vi "Add PV (NT Enum (Index & Choices)).vi"(6 "initial timestamp":timestamp, 7 "PV name":string, 8 "error in (no error)":errorcluster, 9 "initial choices":string[](array[string]), 10 "initial index":u16(ring), 11 "Server in":refnum<class "Server.lvclass">) -> (0 "error out":errorcluster, 1 "choices out":string[](array[string]), 2 "value out":u16, 3 "Server out":refnum<class "Server.lvclass">, 4 "timestamp out":timestamp)   [LabVIEW 2020, in "PV Access.lvlib" / "PVA Server.lvlib" / "Server.lvclass"]
uses:
  Server.lvclass
  PV Data/NT Enum/NT Enum.lvclass
  C:/Users/eyw68381/source/repos/pvaccess-labview/labview/source/PV Data/NT Base/NT Base.lvclass
  Source/Source.lvclass
  PV Data/PV Data.lvlib
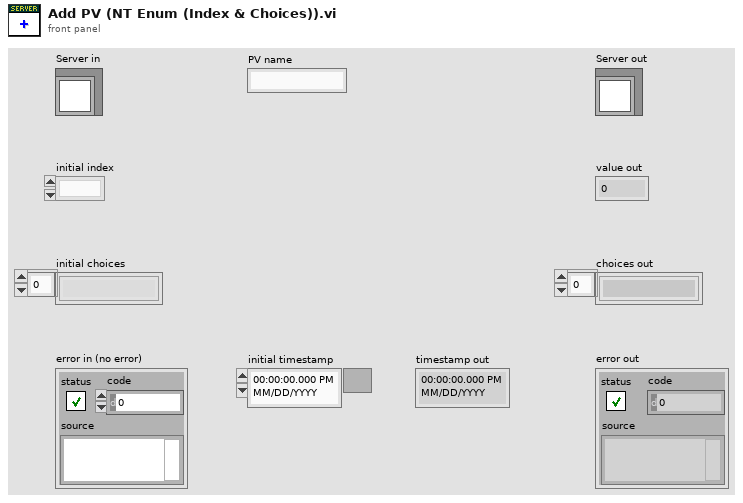
[diagram p1: front panel]
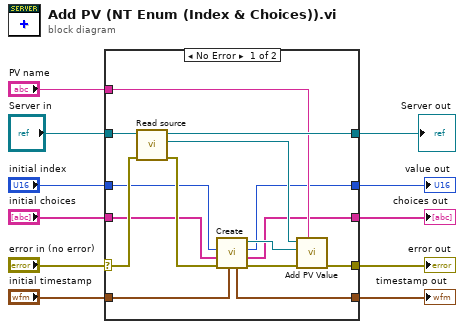
[diagram p0: block diagram]
diagram:
  n1 = case shown="No Error" "error in (no error)" {
    selector: "error in (no error)" -> [w22 w31]
    tunnel: [w21 w31] -> w10
    tunnel: [w25 w30] -> w8
    tunnel: "Server in" -> [w26 w30]
    tunnel: "PV name" -> [w23 _]
    tunnel: "initial index" -> [w17 w29]
    tunnel: [w16 w29] -> w5
    tunnel: "initial timestamp" -> [w15 w28]
    tunnel: [w14 w28] -> w3
    tunnel: "initial choices" -> [w13 w27]
    tunnel: [w12 w27] -> w1
    frame No Error {
      n2 = call "Read source.vi"("error in (no error)"=w22, "Server in"=w26) -> ("error out"=w20:errorcluster, "Source"=w24:refnum<class "Source.lvclass">, "Server out"=w25:refnum<class "Server.lvclass">)  [unwired: 7 in]
      n3 = call-poly "Create.vi"("initial timestamp"=w15, "error in (no error)"=w20, "choices"=w13, "initial index"=w17) -> ("error out"=w19:errorcluster, "choices out"=w12:string[], "index out"=w16:u16, "NT Enum out"=w18:refnum<class "NT Enum.lvclass">, "timestamp out"=w14:timestamp)  [unwired: 3 in]
      n4 = call "Add PV Value.vi"("PV name"=w23, "error in"=w19, "NT Base in"=w18, "Source in"=w24) -> ("error out"=w21:errorcluster)  [unwired: 5 in, 2 out]
    }
    frame Error {
    }
  }
  "error out" <- w10
  "Server out" <- w8
  "value out" <- w5
  "timestamp out" <- w3
  "choices out" <- w1
